vi "State_Machine.vi"(8 "error in (no error)":errorcluster caption="entrée d'erreur (pas d'erreur)", 11 "Get_Voltage en entrée":refnum<class "Nodon_Start_ZCR.lvclass">) -> (0 "error out":errorcluster caption="sortie d'erreur", 2 "Json_String":string, 3 "Get_Voltage en sortie":refnum<class "Nodon_Start_ZCR.lvclass">)   [LabVIEW 2020, in "Library Test.lvlib" / "Nodon_Start_ZCR.lvclass"]
uses:
  Nodon_Start_ZCR.lvclass
  C:/Users/ngarcin/OneDrive - Altyor/Standard TB/Suite TB45/Class/Test/Test (Default)/Test (Default).lvclass
  C:/Users/ngarcin/OneDrive - Altyor/Standard TB/Suite TB45/Class/Test/Nodon_Send_Command_UART/Nodon_Send_Command_UART.lvclass
  Commun VI/TypeDef/Variable Printable.ctl
  JSON API/JSON Value/Set from JSON string.vi
  JSON API/JSON Value/JSON Value.lvclass
  Nodon_Send_Command_UART/Nodon_Send_Command_UART.lvclass
  JSON API/Variant JSON/Variant JSON.lvlib
  JSON API/Get Polymorphic/JSON GetSet.lvlib
  Commun VI/Library Commun.lvlib
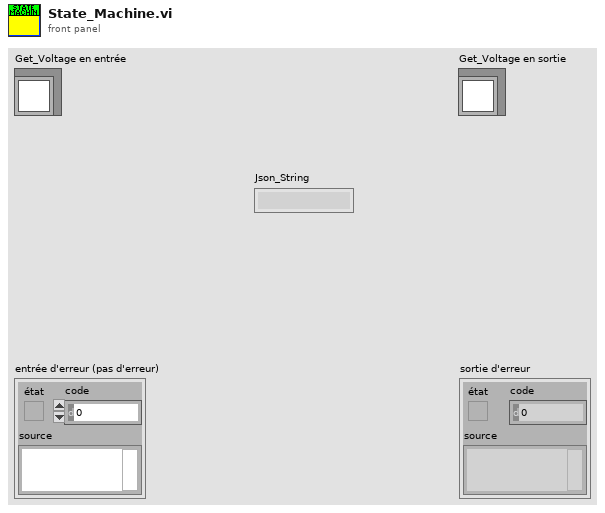
[diagram p1: front panel]
types:
  T1 = cluster{"Channel":string, "Action":string, "Controle_ZCR":bool}
  T2 = typedef "Variable Printable.ctl" = string
  T3 = enum16{"Get Variable", "Get All Variables", "Set Variable", "Delete Variable", "Delete All Variable"}
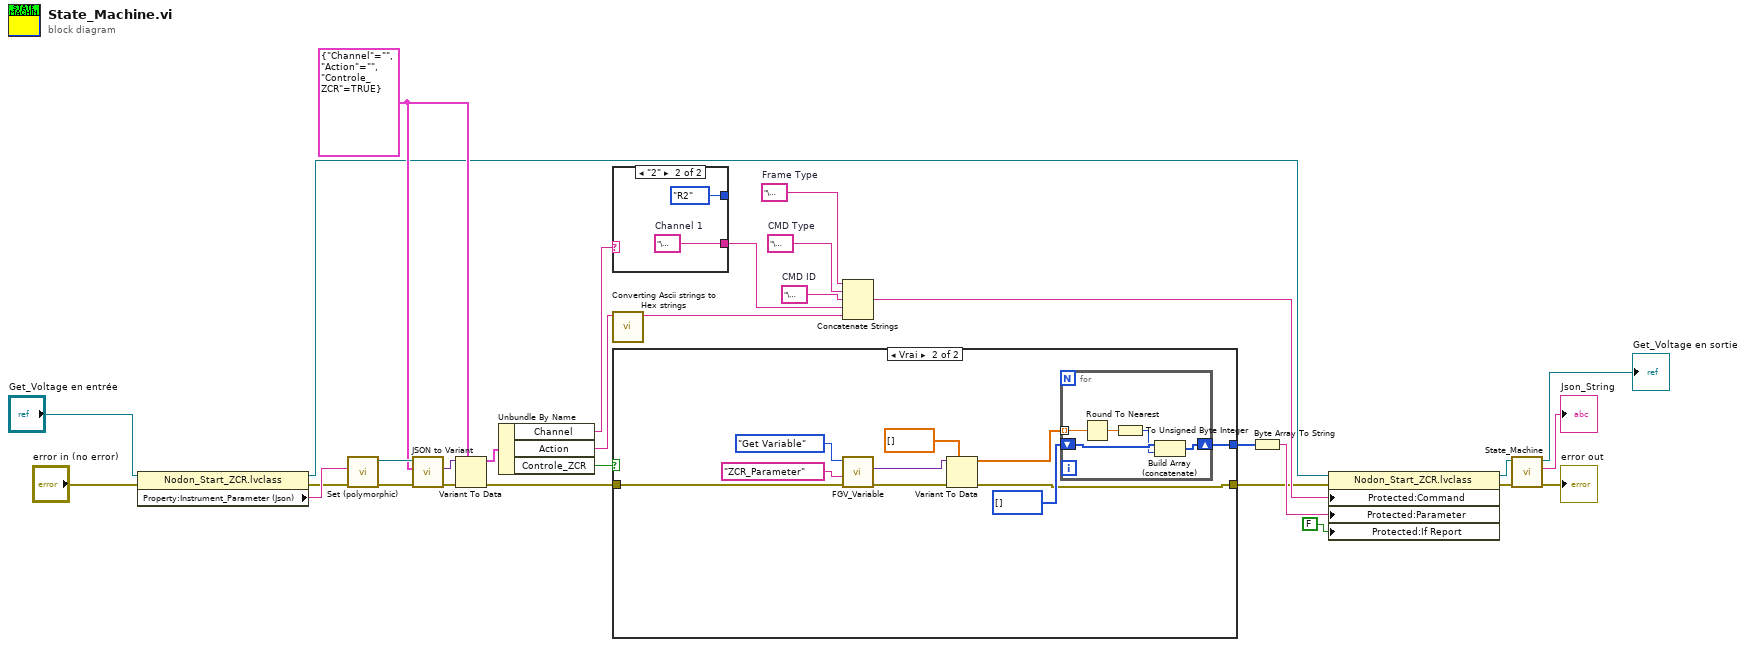
[diagram p0: block diagram]
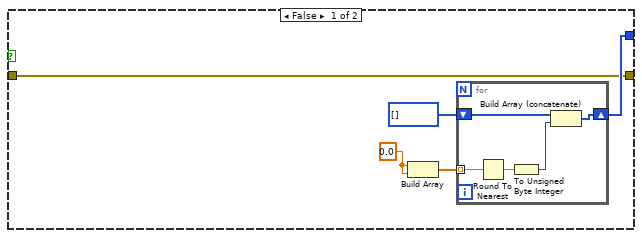
[diagram p2: hidden frame]
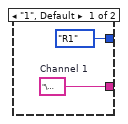
[diagram p3: hidden frame]
diagram:
  w12 = T1 {"Channel"="", "Action"="", "Controle_ZCR"=TRUE}
  w25 = "\u0000"  # Frame Type
  w24 = "\u0000"  # CMD ID
  w23 = "\u0003"  # CMD Type
  n1 = property class="Nodon_Start_ZCR.lvclass"(reference="Get_Voltage en entrée", error in="error in (no error)") -> (reference out=w6:refnum<class "Nodon_Start_ZCR.lvclass">, error out=w13:errorcluster, "Property:Instrument_Parameter (Json)"=w14:string)
  n2 = call-poly "Set (polymorphic).vi"("error in (no error)"=w13, "JSON stream"=w14) -> ("error out"=w16:errorcluster, "JSON Value out"=w18:refnum<class "JSON Value.lvclass">)  [unwired: 7 in, 1 out]
  n3 = call "JSON to Variant.vi"("error in (no error)"=w16, "Variant (Data Type)"=w12, "JSON Value"=w18) -> ("error out"=w17:errorcluster, "Variant out"=w15:variant)  [unwired: 7 in]
  n4 = Variant To Data(error in=w17, type=w12, Variant=w15) -> (data=w11:T1, error out=w2:errorcluster)
  n5 = Unbundle By Name(w11) -> ("Channel"=w8:string, "Action"=w5:string, "Controle_ZCR"=w3:bool)
  n6 = case shown="\"2\"" w8 {
    tunnel: [enum16{"R1", "R2"}."R1" ("Relay") enum16{"R1", "R2"}."R2" ("Relay")] -> _
    tunnel: [w31 w33] -> w7
    frame "1", Default {
      w31 = "\u0000"  # Channel 1
    }
    frame "2" {
      w33 = "\u0001"  # Channel 1
    }
  }
  n7 = call "Converting Ascii strings to Hex strings.vi"("result string"=w5) -> ("Chaîne"=w4:string)  [unwired: 10 in]
  n8 = case shown="Vrai" w3 {
    tunnel: [w37 w53] -> w20
    tunnel: w2 -> [w35 w47]
    tunnel: [w35 w46] -> w1
    frame False {
      w36 = 0.0 ("élément")
      n9 = Build Array(w36, w36) -> (w38:dbl[])
      n10 = for {
        shift-right: [w44] -> w37
        shift-left: u8[] [] -> [w43]
        tunnel: w38 -> [w42] mode=indexing
        n11 = Round To Nearest(number=w42) -> (nearest integer value=w40:dbl)
        n12 = To Unsigned Byte Integer(number=w40) -> (unsigned 8bit integer=w41:u8)
        n13 = Build Array (concatenate)(w43, w41) -> (w44:u8[])
      }
    }
    frame True {
      n14 = call "FGV_Variable.vi"("error in (no error)"=w47, "Variable"=T2 "ZCR_Parameter", "Function"=T3."Get Variable") -> ("error out"=w48:errorcluster, "Data Out"=w50:variant)  [unwired: 6 in, 1 out]
      n15 = Variant To Data(error in=w48, type=dbl[] [] ("tableau ajouté"), Variant=w50) -> (data=w45:dbl[], error out=w46:errorcluster)
      n16 = for {
        shift-right: [w59] -> w53
        shift-left: u8[] [] -> [w58]
        tunnel: w45 -> [w57] mode=indexing
        n17 = Round To Nearest(number=w57) -> (nearest integer value=w55:dbl)
        n18 = To Unsigned Byte Integer(number=w55) -> (unsigned 8bit integer=w56:u8)
        n19 = Build Array (concatenate)(w58, w56) -> (w59:u8[])
      }
    }
  }
  n20 = Concatenate Strings(w25, w23, w24, w7, w4) -> (w22:string)
  n21 = Byte Array To String(unsigned byte array=w20) -> (string=w19:string)
  n22 = property class="Nodon_Start_ZCR.lvclass"(reference=w6, error in=w1, "Protected:Command"=w22, "Protected:Parameter"=w19, "Protected:If Report"=FALSE ("If Report")) -> (reference out=w27:refnum<class "Nodon_Start_ZCR.lvclass">, error out=w26:errorcluster)
  n23 = call-parent "State_Machine.vi"("error in (no error)"=w26, "Send_Frame en entrée"=w27) -> ("error out"=→"error out":errorcluster, "Json_String"=→"Json_String":string, "Send_Frame en sortie"=→"Get_Voltage en sortie":refnum<class "Nodon_Start_ZCR.lvclass">)  [unwired: 7 in]
